vi "Get Data.vi"(7 "?":T1={"Input Data 1D"=[], "Channel Settings"={"Supply Voltage [Vdc]"=0.0, "Max Supply Current [Idc]"=0.0, "Settling Delay"=0.0, "Temp Criteria"=0.0, "Voltage Steps [Vrms]"=[0.0, 0.25, 0.5, 1.0, 1.95, 3.0, 3.9, 5.5], "User Notes"="", "Config Wave File Path"=path "C:/ASD Power Point Beta 32J/Waveforms/150HzSine5Second.wav", "Config Voltage [Vrms]"=0.0, "Channel Configuration List"={"Channel Configuration Cluster"={"Input"=enum."---", "Enable"=FALSE, "User Notes"="", "Voltage Range"=0.0, "Current Range"=2.5}, "Channel Configuration Cluster 2"={"Input"=enum."---", "Enable"=FALSE, "User Notes"="", "Voltage Range"=0.0, "Current Range"=2.5}, "Channel Configuration Cluster 3"={"Input"=enum."---", "Enable"=FALSE, "User Notes"="", "Voltage Range"=0.0, "Current Range"=2.5}, "Channel Configuration Cluster 4"={"Input"=enum."---", "Enable"=FALSE, "User Notes"="", "Voltage Range"=0.0, "Current Range"=2.5}, "Channel Configuration Cluster 5"={"Input"=enum."---", "Enable"=FALSE, "User Notes"="", "Voltage Range"=0.0, "Current Range"=2.5}, "Channel Configuration Cluster 6"={"Input"=enum."---", "Enable"=FALSE, "User Notes"="", "Voltage Range"=0.0, "Current Range"=2.5}, "Channel Configuration Cluster 7"={"Input"=enum."---", "Enable"=FALSE, "User Notes"="", "Voltage Range"=0.0, "Current Range"=2.5}, "Channel Configuration Cluster 8"={"Input"=enum."---", "Enable"=FALSE, "User Notes"="", "Voltage Range"=0.0, "Current Range"=2.5}, "Channel Configuration Cluster 9"={"Input"=enum."---", "Enable"=FALSE, "User Notes"="", "Voltage Range"=0.0, "Current Range"=2.5}, "Channel Configuration Cluster 10"={"Input"=enum."---", "Enable"=FALSE, "User Notes"="", "Voltage Range"=0.0, "Current Range"=2.5}, "Channel Configuration Cluster 11"={"Input"=enum."---", "Enable"=FALSE, "User Notes"="", "Voltage Range"=0.0, "Current Range"=2.5}, "Channel Configuration Cluster 12"={"Input"=enum."---", "Enable"=FALSE, "User Notes"="", "Voltage Range"=0.0, "Current Range"=2.5}, "Channel Configuration Cluster 13"={"Input"=enum."---", "Enable"=FALSE, "User Notes"="", "Voltage Range"=0.0, "Current Range"=2.5}, "Channel Configuration Cluster 14"={"Input"=enum."---", "Enable"=FALSE, "User Notes"="", "Voltage Range"=0.0, "Current Range"=2.5}, "Channel Configuration Cluster 15"={"Input"=enum."---", "Enable"=FALSE, "User Notes"="", "Voltage Range"=0.0, "Current Range"=2.5}, "Channel Configuration Cluster 16"={"Input"=enum."---", "Enable"=FALSE, "User Notes"="", "Voltage Range"=0.0, "Current Range"=2.5}, "Channel Configuration Cluster 17"={"Input"=enum."---", "Enable"=FALSE, "User Notes"="", "Voltage Range"=0.0, "Current Range"=2.5}}, "User Gains"={"Gain 1"=0.0, "Gain 2"=0.0, "Gain 3"=0.0, "Gain 4"=0.0, "Gain 5"=0.0, "Gain 6"=0.0}, "Gains"={"Gain 1"=0.0, "Gain 2"=0.0, "Gain 3"=0.0, "Gain 4"=0.0, "Gain 5"=0.0, "Gain 6"=0.0}, "Gain Array"={"Gain 1"=0.0, "Gain 2"=0.0, "Gain 3"=0.0, "Gain 4"=0.0, "Gain 5"=0.0, "Gain 6"=0.0, "Gain 7"=0.0, "Gain 8"=0.0, "Gain 9"=0.0, "Gain 10"=0.0, "Gain 11"=0.0, "Gain 12"=0.0, "Gain 13"=0.0, "Gain 14"=0.0, "Gain 15"=0.0, "Gain 16"=0.0, "Gain 17"=0.0}, "Wave File Path 1"=path "", "Wave File Path 2"=path "", "Wave File Path 3"=path "", "Wave File Path 4"=path "", "Range"=FALSE, "CF"=FALSE}, "Select Data"={"Vrms Data"=FALSE, "Vpkpk Data"=FALSE, "Irms Data"=FALSE, "Power Data"=FALSE, "Ipkpk Data"=FALSE, "Temp Data"=FALSE}, "Detailed Report ?"=FALSE, "Path Settings:"={"Template Path "=path "E:/L&T Projects/Bose ASD/Excel Template/ASD Template.xltx", "Report Path"=path "E:/L&T Projects/Bose ASD/excel Reports", "JPEG1 Path "=path "C:/Users/Public/Pictures/Sample Pictures/Hydrangeas.jpg", "JPEG2 Path"=path "C:/Users/Public/Pictures/Sample Pictures/Lighthouse.jpg"}, "Vrms_Sheet"=[], "Irms_Sheet"=[], "Power_Sheet"=[], "Vpk_Sheet"=[], "Ipk_Sheet"=[], "Vrms_Avg"=[], "Irms_Avg"=[], "Power_Avg"=[], "Vpk_Avg"=[], "Ipk_Avg"=[], "Report_Ref"=refnum, "User Name"="", "Temp_Sheet"=[]} {"Channel Settings"."Gain Array"."Gain 17" format="%.2f"; "Channel Settings"."Gain Array"."Gain 16" format="%.2f"; "Channel Settings"."Gain Array"."Gain 15" format="%.2f"; "Channel Settings"."Gain Array"."Gain 14" format="%.2f"; "Channel Settings"."Gain Array"."Gain 13" format="%.2f"; "Channel Settings"."Gain Array"."Gain 12" format="%.2f"; "Channel Settings"."Gain Array"."Gain 11" format="%.2f"; "Channel Settings"."Gain Array"."Gain 10" format="%.2f"; "Channel Settings"."Gain Array"."Gain 9" format="%.2f"; "Channel Settings"."Gain Array"."Gain 8" format="%.2f"; "Channel Settings"."Gain Array"."Gain 7" format="%.2f"; "Channel Settings"."Gain Array"."Gain 6" format="%.2f"; "Channel Settings"."Gain Array"."Gain 5" format="%.2f"; "Channel Settings"."Gain Array"."Gain 4" format="%.2f"; "Channel Settings"."Gain Array"."Gain 3" format="%.2f"; "Channel Settings"."Gain Array"."Gain 2" format="%.2f"; "Channel Settings"."Gain Array"."Gain 1" format="%.2f"; "Channel Settings"."Gains"."Gain 6" format="%.2f"; "Channel Settings"."Gains"."Gain 5" format="%.2f"; "Channel Settings"."Gains"."Gain 4" format="%.2f"; "Channel Settings"."Gains"."Gain 3" format="%.2f"; "Channel Settings"."Gains"."Gain 2" format="%.2f"; "Channel Settings"."Gains"."Gain 1" format="%.2f"; "Channel Settings"."User Gains"."Gain 6" format="%.2f"; "Channel Settings"."User Gains"."Gain 5" format="%.2f"; "Channel Settings"."User Gains"."Gain 4" format="%.2f"; "Channel Settings"."User Gains"."Gain 3" format="%.2f"; "Channel Settings"."User Gains"."Gain 2" format="%.2f"; "Channel Settings"."User Gains"."Gain 1" format="%.2f"; "Channel Settings"."Channel Configuration List"."Channel Configuration Cluster 17"."Current Range" items=["1 <500m>"=0.5, "2 <1>"=1.0, "5 <2.5>"=2.5, "10 <5>"=5.0, "20 <10>"=10.0, "50 <25>"=25.0]; "Channel Settings"."Channel Configuration List"."Channel Configuration Cluster 17"."Voltage Range" items=["1.5 <0.75>"=0.75, "3 <1.5>"=1.5, "6 <3>"=3.0, "10 <5>"=5.0, "15 <7.5>"=7.5, "30 <15>"=15.0, "60 <30>"=30.0, "100 <50>"=50.0, "150 <75>"=75.0, "300 <150>"=150.0, "600 <300>"=300.0, "1000 <500>"=500.0]; "Channel Settings"."Channel Configuration List"."Channel Configuration Cluster 16"."Current Range" items=["1 <500m>"=0.5, "2 <1>"=1.0, "5 <2.5>"=2.5, "10 <5>"=5.0, "20 <10>"=10.0, "50 <25>"=25.0]; "Channel Settings"."Channel Configuration List"."Channel Configuration Cluster 16"."Voltage Range" items=["1.5 <0.75>"=0.75, "3 <1.5>"=1.5, "6 <3>"=3.0, "10 <5>"=5.0, "15 <7.5>"=7.5, "30 <15>"=15.0, "60 <30>"=30.0, "100 <50>"=50.0, "150 <75>"=75.0, "300 <150>"=150.0, "600 <300>"=300.0, "1000 <500>"=500.0]; "Channel Settings"."Channel Configuration List"."Channel Configuration Cluster 15"."Current Range" items=["1 <500m>"=0.5, "2 <1>"=1.0, "5 <2.5>"=2.5, "10 <5>"=5.0, "20 <10>"=10.0, "50 <25>"=25.0]; "Channel Settings"."Channel Configuration List"."Channel Configuration Cluster 15"."Voltage Range" items=["1.5 <0.75>"=0.75, "3 <1.5>"=1.5, "6 <3>"=3.0, "10 <5>"=5.0, "15 <7.5>"=7.5, "30 <15>"=15.0, "60 <30>"=30.0, "100 <50>"=50.0, "150 <75>"=75.0, "300 <150>"=150.0, "600 <300>"=300.0, "1000 <500>"=500.0]; "Channel Settings"."Channel Configuration List"."Channel Configuration Cluster 14"."Current Range" items=["1 <500m>"=0.5, "2 <1>"=1.0, "5 <2.5>"=2.5, "10 <5>"=5.0, "20 <10>"=10.0, "50 <25>"=25.0]; "Channel Settings"."Channel Configuration List"."Channel Configuration Cluster 14"."Voltage Range" items=["1.5 <0.75>"=0.75, "3 <1.5>"=1.5, "6 <3>"=3.0, "10 <5>"=5.0, "15 <7.5>"=7.5, "30 <15>"=15.0, "60 <30>"=30.0, "100 <50>"=50.0, "150 <75>"=75.0, "300 <150>"=150.0, "600 <300>"=300.0, "1000 <500>"=500.0]; "Channel Settings"."Channel Configuration List"."Channel Configuration Cluster 13"."Current Range" items=["1 <500m>"=0.5, "2 <1>"=1.0, "5 <2.5>"=2.5, "10 <5>"=5.0, "20 <10>"=10.0, "50 <25>"=25.0]; "Channel Settings"."Channel Configuration List"."Channel Configuration Cluster 13"."Voltage Range" items=["1.5 <0.75>"=0.75, "3 <1.5>"=1.5, "6 <3>"=3.0, "10 <5>"=5.0, "15 <7.5>"=7.5, "30 <15>"=15.0, "60 <30>"=30.0, "100 <50>"=50.0, "150 <75>"=75.0, "300 <150>"=150.0, "600 <300>"=300.0, "1000 <500>"=500.0]; "Channel Settings"."Channel Configuration List"."Channel Configuration Cluster 12"."Current Range" items=["1 <500m>"=0.5, "2 <1>"=1.0, "5 <2.5>"=2.5, "10 <5>"=5.0, "20 <10>"=10.0, "50 <25>"=25.0]; "Channel Settings"."Channel Configuration List"."Channel Configuration Cluster 12"."Voltage Range" items=["1.5 <0.75>"=0.75, "3 <1.5>"=1.5, "6 <3>"=3.0, "10 <5>"=5.0, "15 <7.5>"=7.5, "30 <15>"=15.0, "60 <30>"=30.0, "100 <50>"=50.0, "150 <75>"=75.0, "300 <150>"=150.0, "600 <300>"=300.0, "1000 <500>"=500.0]; "Channel Settings"."Channel Configuration List"."Channel Configuration Cluster 11"."Current Range" items=["1 <500m>"=0.5, "2 <1>"=1.0, "5 <2.5>"=2.5, "10 <5>"=5.0, "20 <10>"=10.0, "50 <25>"=25.0]; "Channel Settings"."Channel Configuration List"."Channel Configuration Cluster 11"."Voltage Range" items=["1.5 <0.75>"=0.75, "3 <1.5>"=1.5, "6 <3>"=3.0, "10 <5>"=5.0, "15 <7.5>"=7.5, "30 <15>"=15.0, "60 <30>"=30.0, "100 <50>"=50.0, "150 <75>"=75.0, "300 <150>"=150.0, "600 <300>"=300.0, "1000 <500>"=500.0]; "Channel Settings"."Channel Configuration List"."Channel Configuration Cluster 10"."Current Range" items=["1 <500m>"=0.5, "2 <1>"=1.0, "5 <2.5>"=2.5, "10 <5>"=5.0, "20 <10>"=10.0, "50 <25>"=25.0]; "Channel Settings"."Channel Configuration List"."Channel Configuration Cluster 10"."Voltage Range" items=["1.5 <0.75>"=0.75, "3 <1.5>"=1.5, "6 <3>"=3.0, "10 <5>"=5.0, "15 <7.5>"=7.5, "30 <15>"=15.0, "60 <30>"=30.0, "100 <50>"=50.0, "150 <75>"=75.0, "300 <150>"=150.0, "600 <300>"=300.0, "1000 <500>"=500.0]; "Channel Settings"."Channel Configuration List"."Channel Configuration Cluster 9"."Voltage Range" items=["1.5 <0.75>"=0.75, "3 <1.5>"=1.5, "6 <3>"=3.0, "10 <5>"=5.0, "15 <7.5>"=7.5, "30 <15>"=15.0, "60 <30>"=30.0, "100 <50>"=50.0, "150 <75>"=75.0, "300 <150>"=150.0, "600 <300>"=300.0, "1000 <500>"=500.0]; "Channel Settings"."Channel Configuration List"."Channel Configuration Cluster 9"."Current Range" items=["10m <5m>"=0.005, "20m <10m>"=0.01, "50m <25m>"=0.025, "100m <50m>"=0.05, "200m <100m>"=0.1, "500m <250m>"=0.25, "1 <500m>"=0.5, "2 <1>"=1.0, "5 <2.5>"=2.5]; "Channel Settings"."Channel Configuration List"."Channel Configuration Cluster 8"."Voltage Range" items=["1.5 <0.75>"=0.75, "3 <1.5>"=1.5, "6 <3>"=3.0, "10 <5>"=5.0, "15 <7.5>"=7.5, "30 <15>"=15.0, "60 <30>"=30.0, "100 <50>"=50.0, "150 <75>"=75.0, "300 <150>"=150.0, "600 <300>"=300.0, "1000 <500>"=500.0]; "Channel Settings"."Channel Configuration List"."Channel Configuration Cluster 8"."Current Range" items=["10m <5m>"=0.005, "20m <10m>"=0.01, "50m <25m>"=0.025, "100m <50m>"=0.05, "200m <100m>"=0.1, "500m <250m>"=0.25, "1 <500m>"=0.5, "2 <1>"=1.0, "5 <2.5>"=2.5]; "Channel Settings"."Channel Configuration List"."Channel Configuration Cluster 7"."Voltage Range" items=["1.5 <0.75>"=0.75, "3 <1.5>"=1.5, "6 <3>"=3.0, "10 <5>"=5.0, "15 <7.5>"=7.5, "30 <15>"=15.0, "60 <30>"=30.0, "100 <50>"=50.0, "150 <75>"=75.0, "300 <150>"=150.0, "600 <300>"=300.0, "1000 <500>"=500.0]; "Channel Settings"."Channel Configuration List"."Channel Configuration Cluster 7"."Current Range" items=["10m <5m>"=0.005, "20m <10m>"=0.01, "50m <25m>"=0.025, "100m <50m>"=0.05, "200m <100m>"=0.1, "500m <250m>"=0.25, "1 <500m>"=0.5, "2 <1>"=1.0, "5 <2.5>"=2.5]; "Channel Settings"."Channel Configuration List"."Channel Configuration Cluster 6"."Voltage Range" items=["1.5 <0.75>"=0.75, "3 <1.5>"=1.5, "6 <3>"=3.0, "10 <5>"=5.0, "15 <7.5>"=7.5, "30 <15>"=15.0, "60 <30>"=30.0, "100 <50>"=50.0, "150 <75>"=75.0, "300 <150>"=150.0, "600 <300>"=300.0, "1000 <500>"=500.0]; "Channel Settings"."Channel Configuration List"."Channel Configuration Cluster 6"."Current Range" items=["10m <5m>"=0.005, "20m <10m>"=0.01, "50m <25m>"=0.025, "100m <50m>"=0.05, "200m <100m>"=0.1, "500m <250m>"=0.25, "1 <500m>"=0.5, "2 <1>"=1.0, "5 <2.5>"=2.5]; "Channel Settings"."Channel Configuration List"."Channel Configuration Cluster 5"."Voltage Range" items=["1.5 <0.75>"=0.75, "3 <1.5>"=1.5, "6 <3>"=3.0, "10 <5>"=5.0, "15 <7.5>"=7.5, "30 <15>"=15.0, "60 <30>"=30.0, "100 <50>"=50.0, "150 <75>"=75.0, "300 <150>"=150.0, "600 <300>"=300.0, "1000 <500>"=500.0]; "Channel Settings"."Channel Configuration List"."Channel Configuration Cluster 5"."Current Range" items=["10m <5m>"=0.005, "20m <10m>"=0.01, "50m <25m>"=0.025, "100m <50m>"=0.05, "200m <100m>"=0.1, "500m <250m>"=0.25, "1 <500m>"=0.5, "2 <1>"=1.0, "5 <2.5>"=2.5]; "Channel Settings"."Channel Configuration List"."Channel Configuration Cluster 4"."Voltage Range" items=["1.5 <0.75>"=0.75, "3 <1.5>"=1.5, "6 <3>"=3.0, "10 <5>"=5.0, "15 <7.5>"=7.5, "30 <15>"=15.0, "60 <30>"=30.0, "100 <50>"=50.0, "150 <75>"=75.0, "300 <150>"=150.0, "600 <300>"=300.0, "1000 <500>"=500.0]; "Channel Settings"."Channel Configuration List"."Channel Configuration Cluster 4"."Current Range" items=["10m <5m>"=0.005, "20m <10m>"=0.01, "50m <25m>"=0.025, "100m <50m>"=0.05, "200m <100m>"=0.1, "500m <250m>"=0.25, "1 <500m>"=0.5, "2 <1>"=1.0, "5 <2.5>"=2.5]; "Channel Settings"."Channel Configuration List"."Channel Configuration Cluster 3"."Voltage Range" items=["1.5 <0.75>"=0.75, "3 <1.5>"=1.5, "6 <3>"=3.0, "10 <5>"=5.0, "15 <7.5>"=7.5, "30 <15>"=15.0, "60 <30>"=30.0, "100 <50>"=50.0, "150 <75>"=75.0, "300 <150>"=150.0, "600 <300>"=300.0, "1000 <500>"=500.0]; "Channel Settings"."Channel Configuration List"."Channel Configuration Cluster 3"."Current Range" items=["10m <5m>"=0.005, "20m <10m>"=0.01, "50m <25m>"=0.025, "100m <50m>"=0.05, "200m <100m>"=0.1, "500m <250m>"=0.25, "1 <500m>"=0.5, "2 <1>"=1.0, "5 <2.5>"=2.5]; "Channel Settings"."Channel Configuration List"."Channel Configuration Cluster 2"."Voltage Range" items=["1.5 <0.75>"=0.75, "3 <1.5>"=1.5, "6 <3>"=3.0, "10 <5>"=5.0, "15 <7.5>"=7.5, "30 <15>"=15.0, "60 <30>"=30.0, "100 <50>"=50.0, "150 <75>"=75.0, "300 <150>"=150.0, "600 <300>"=300.0, "1000 <500>"=500.0]; "Channel Settings"."Channel Configuration List"."Channel Configuration Cluster 2"."Current Range" items=["10m <5m>"=0.005, "20m <10m>"=0.01, "50m <25m>"=0.025, "100m <50m>"=0.05, "200m <100m>"=0.1, "500m <250m>"=0.25, "1 <500m>"=0.5, "2 <1>"=1.0, "5 <2.5>"=2.5]; "Channel Settings"."Channel Configuration List"."Channel Configuration Cluster"."Voltage Range" items=["1.5 <0.75>"=0.75, "3 <1.5>"=1.5, "6 <3>"=3.0, "10 <5>"=5.0, "15 <7.5>"=7.5, "30 <15>"=15.0, "60 <30>"=30.0, "100 <50>"=50.0, "150 <75>"=75.0, "300 <150>"=150.0, "600 <300>"=300.0, "1000 <500>"=500.0]; "Channel Settings"."Channel Configuration List"."Channel Configuration Cluster"."Current Range" items=["10m <5m>"=0.005, "20m <10m>"=0.01, "50m <25m>"=0.025, "100m <50m>"=0.05, "200m <100m>"=0.1, "500m <250m>"=0.25, "1 <500m>"=0.5, "2 <1>"=1.0, "5 <2.5>"=2.5]; "Channel Settings"."Settling Delay" min=0.0 format="%<%H:%M:%S>t"; "Input Data 1D"."WT1800 Averages"."Vrms" format="%.3f"; "Input Data 1D"."WT1800 Averages"."Irms" format="%.3f"; "Input Data 1D"."WT1800 Averages"."Power" format="%.3f"; "Input Data 1D"."WT1800 Averages"."Vpkpk" format="%.3f"; "Input Data 1D"."WT1800 Averages"."Ipkpk" format="%.3f"; "Input Data 1D"."WT1800 Measurements"."Vrms" format="%.3f"; "Input Data 1D"."WT1800 Measurements"."Irms" format="%.3f"; "Input Data 1D"."WT1800 Measurements"."Power" format="%.3f"; "Input Data 1D"."WT1800 Measurements"."Vpkpk" format="%.3f"; "Input Data 1D"."WT1800 Measurements"."Ipkpk" format="%.3f"; "Input Data 1D"."DSA Averages"."Vrms" format="%.3f"; "Input Data 1D"."DSA Averages"."Vdc" format="%.3f"; "Input Data 1D"."DSA Averages"."Vpk+" format="%.3f"; "Input Data 1D"."DSA Averages"."Vpk-" format="%.3f"; "Input Data 1D"."DSA Averages"."Vpkpk" format="%.3f"; "Input Data 1D"."DSA Measurements"."Vrms" format="%.3f"; "Input Data 1D"."DSA Measurements"."Vdc" format="%.3f"; "Input Data 1D"."DSA Measurements"."Vpk+" format="%.3f"; "Input Data 1D"."DSA Measurements"."Vpk-" format="%.3f"; "Input Data 1D"."DSA Measurements"."Vpkpk" format="%.3f"}, 8 "error in":errorcluster) -> (0 "error out":errorcluster, 5 "output cluster":T1={"Input Data 1D"=[], "Channel Settings"={"Supply Voltage [Vdc]"=0.0, "Max Supply Current [Idc]"=0.0, "Settling Delay"=0.0, "Temp Criteria"=0.0, "Voltage Steps [Vrms]"=[0.0, 0.25, 0.5, 1.0, 1.95, 3.0, 3.9, 5.5], "User Notes"="", "Config Wave File Path"=path "C:/ASD Power Point Beta 32J/Waveforms/150HzSine5Second.wav", "Config Voltage [Vrms]"=0.0, "Channel Configuration List"={"Channel Configuration Cluster"={"Input"=enum."---", "Enable"=FALSE, "User Notes"="", "Voltage Range"=0.0, "Current Range"=2.5}, "Channel Configuration Cluster 2"={"Input"=enum."---", "Enable"=FALSE, "User Notes"="", "Voltage Range"=0.0, "Current Range"=2.5}, "Channel Configuration Cluster 3"={"Input"=enum."---", "Enable"=FALSE, "User Notes"="", "Voltage Range"=0.0, "Current Range"=2.5}, "Channel Configuration Cluster 4"={"Input"=enum."---", "Enable"=FALSE, "User Notes"="", "Voltage Range"=0.0, "Current Range"=2.5}, "Channel Configuration Cluster 5"={"Input"=enum."---", "Enable"=FALSE, "User Notes"="", "Voltage Range"=0.0, "Current Range"=2.5}, "Channel Configuration Cluster 6"={"Input"=enum."---", "Enable"=FALSE, "User Notes"="", "Voltage Range"=0.0, "Current Range"=2.5}, "Channel Configuration Cluster 7"={"Input"=enum."---", "Enable"=FALSE, "User Notes"="", "Voltage Range"=0.0, "Current Range"=2.5}, "Channel Configuration Cluster 8"={"Input"=enum."---", "Enable"=FALSE, "User Notes"="", "Voltage Range"=0.0, "Current Range"=2.5}, "Channel Configuration Cluster 9"={"Input"=enum."---", "Enable"=FALSE, "User Notes"="", "Voltage Range"=0.0, "Current Range"=2.5}, "Channel Configuration Cluster 10"={"Input"=enum."---", "Enable"=FALSE, "User Notes"="", "Voltage Range"=0.0, "Current Range"=2.5}, "Channel Configuration Cluster 11"={"Input"=enum."---", "Enable"=FALSE, "User Notes"="", "Voltage Range"=0.0, "Current Range"=2.5}, "Channel Configuration Cluster 12"={"Input"=enum."---", "Enable"=FALSE, "User Notes"="", "Voltage Range"=0.0, "Current Range"=2.5}, "Channel Configuration Cluster 13"={"Input"=enum."---", "Enable"=FALSE, "User Notes"="", "Voltage Range"=0.0, "Current Range"=2.5}, "Channel Configuration Cluster 14"={"Input"=enum."---", "Enable"=FALSE, "User Notes"="", "Voltage Range"=0.0, "Current Range"=2.5}, "Channel Configuration Cluster 15"={"Input"=enum."---", "Enable"=FALSE, "User Notes"="", "Voltage Range"=0.0, "Current Range"=2.5}, "Channel Configuration Cluster 16"={"Input"=enum."---", "Enable"=FALSE, "User Notes"="", "Voltage Range"=0.0, "Current Range"=2.5}, "Channel Configuration Cluster 17"={"Input"=enum."---", "Enable"=FALSE, "User Notes"="", "Voltage Range"=0.0, "Current Range"=2.5}}, "User Gains"={"Gain 1"=0.0, "Gain 2"=0.0, "Gain 3"=0.0, "Gain 4"=0.0, "Gain 5"=0.0, "Gain 6"=0.0}, "Gains"={"Gain 1"=0.0, "Gain 2"=0.0, "Gain 3"=0.0, "Gain 4"=0.0, "Gain 5"=0.0, "Gain 6"=0.0}, "Gain Array"={"Gain 1"=0.0, "Gain 2"=0.0, "Gain 3"=0.0, "Gain 4"=0.0, "Gain 5"=0.0, "Gain 6"=0.0, "Gain 7"=0.0, "Gain 8"=0.0, "Gain 9"=0.0, "Gain 10"=0.0, "Gain 11"=0.0, "Gain 12"=0.0, "Gain 13"=0.0, "Gain 14"=0.0, "Gain 15"=0.0, "Gain 16"=0.0, "Gain 17"=0.0}, "Wave File Path 1"=path "", "Wave File Path 2"=path "", "Wave File Path 3"=path "", "Wave File Path 4"=path "", "Range"=FALSE, "CF"=FALSE}, "Select Data"={"Vrms Data"=FALSE, "Vpkpk Data"=FALSE, "Irms Data"=FALSE, "Power Data"=FALSE, "Ipkpk Data"=FALSE, "Temp Data"=FALSE}, "Detailed Report ?"=FALSE, "Path Settings:"={"Template Path "=path "E:/L&T Projects/Bose ASD/Excel Template/ASD Template.xltx", "Report Path"=path "E:/L&T Projects/Bose ASD/excel Reports", "JPEG1 Path "=path "C:/Users/Public/Pictures/Sample Pictures/Hydrangeas.jpg", "JPEG2 Path"=path "C:/Users/Public/Pictures/Sample Pictures/Lighthouse.jpg"}, "Vrms_Sheet"=[], "Irms_Sheet"=[], "Power_Sheet"=[], "Vpk_Sheet"=[], "Ipk_Sheet"=[], "Vrms_Avg"=[], "Irms_Avg"=[], "Power_Avg"=[], "Vpk_Avg"=[], "Ipk_Avg"=[], "Report_Ref"=refnum, "User Name"="", "Temp_Sheet"=[]} {"Channel Settings"."Gain Array"."Gain 17" format="%.2f"; "Channel Settings"."Gain Array"."Gain 16" format="%.2f"; "Channel Settings"."Gain Array"."Gain 15" format="%.2f"; "Channel Settings"."Gain Array"."Gain 14" format="%.2f"; "Channel Settings"."Gain Array"."Gain 13" format="%.2f"; "Channel Settings"."Gain Array"."Gain 12" format="%.2f"; "Channel Settings"."Gain Array"."Gain 11" format="%.2f"; "Channel Settings"."Gain Array"."Gain 10" format="%.2f"; "Channel Settings"."Gain Array"."Gain 9" format="%.2f"; "Channel Settings"."Gain Array"."Gain 8" format="%.2f"; "Channel Settings"."Gain Array"."Gain 7" format="%.2f"; "Channel Settings"."Gain Array"."Gain 6" format="%.2f"; "Channel Settings"."Gain Array"."Gain 5" format="%.2f"; "Channel Settings"."Gain Array"."Gain 4" format="%.2f"; "Channel Settings"."Gain Array"."Gain 3" format="%.2f"; "Channel Settings"."Gain Array"."Gain 2" format="%.2f"; "Channel Settings"."Gain Array"."Gain 1" format="%.2f"; "Channel Settings"."Gains"."Gain 6" format="%.2f"; "Channel Settings"."Gains"."Gain 5" format="%.2f"; "Channel Settings"."Gains"."Gain 4" format="%.2f"; "Channel Settings"."Gains"."Gain 3" format="%.2f"; "Channel Settings"."Gains"."Gain 2" format="%.2f"; "Channel Settings"."Gains"."Gain 1" format="%.2f"; "Channel Settings"."User Gains"."Gain 6" format="%.2f"; "Channel Settings"."User Gains"."Gain 5" format="%.2f"; "Channel Settings"."User Gains"."Gain 4" format="%.2f"; "Channel Settings"."User Gains"."Gain 3" format="%.2f"; "Channel Settings"."User Gains"."Gain 2" format="%.2f"; "Channel Settings"."User Gains"."Gain 1" format="%.2f"; "Channel Settings"."Channel Configuration List"."Channel Configuration Cluster 17"."Current Range" items=["1 <500m>"=0.5, "2 <1>"=1.0, "5 <2.5>"=2.5, "10 <5>"=5.0, "20 <10>"=10.0, "50 <25>"=25.0]; "Channel Settings"."Channel Configuration List"."Channel Configuration Cluster 17"."Voltage Range" items=["1.5 <0.75>"=0.75, "3 <1.5>"=1.5, "6 <3>"=3.0, "10 <5>"=5.0, "15 <7.5>"=7.5, "30 <15>"=15.0, "60 <30>"=30.0, "100 <50>"=50.0, "150 <75>"=75.0, "300 <150>"=150.0, "600 <300>"=300.0, "1000 <500>"=500.0]; "Channel Settings"."Channel Configuration List"."Channel Configuration Cluster 16"."Current Range" items=["1 <500m>"=0.5, "2 <1>"=1.0, "5 <2.5>"=2.5, "10 <5>"=5.0, "20 <10>"=10.0, "50 <25>"=25.0]; "Channel Settings"."Channel Configuration List"."Channel Configuration Cluster 16"."Voltage Range" items=["1.5 <0.75>"=0.75, "3 <1.5>"=1.5, "6 <3>"=3.0, "10 <5>"=5.0, "15 <7.5>"=7.5, "30 <15>"=15.0, "60 <30>"=30.0, "100 <50>"=50.0, "150 <75>"=75.0, "300 <150>"=150.0, "600 <300>"=300.0, "1000 <500>"=500.0]; "Channel Settings"."Channel Configuration List"."Channel Configuration Cluster 15"."Current Range" items=["1 <500m>"=0.5, "2 <1>"=1.0, "5 <2.5>"=2.5, "10 <5>"=5.0, "20 <10>"=10.0, "50 <25>"=25.0]; "Channel Settings"."Channel Configuration List"."Channel Configuration Cluster 15"."Voltage Range" items=["1.5 <0.75>"=0.75, "3 <1.5>"=1.5, "6 <3>"=3.0, "10 <5>"=5.0, "15 <7.5>"=7.5, "30 <15>"=15.0, "60 <30>"=30.0, "100 <50>"=50.0, "150 <75>"=75.0, "300 <150>"=150.0, "600 <300>"=300.0, "1000 <500>"=500.0]; "Channel Settings"."Channel Configuration List"."Channel Configuration Cluster 14"."Current Range" items=["1 <500m>"=0.5, "2 <1>"=1.0, "5 <2.5>"=2.5, "10 <5>"=5.0, "20 <10>"=10.0, "50 <25>"=25.0]; "Channel Settings"."Channel Configuration List"."Channel Configuration Cluster 14"."Voltage Range" items=["1.5 <0.75>"=0.75, "3 <1.5>"=1.5, "6 <3>"=3.0, "10 <5>"=5.0, "15 <7.5>"=7.5, "30 <15>"=15.0, "60 <30>"=30.0, "100 <50>"=50.0, "150 <75>"=75.0, "300 <150>"=150.0, "600 <300>"=300.0, "1000 <500>"=500.0]; "Channel Settings"."Channel Configuration List"."Channel Configuration Cluster 13"."Current Range" items=["1 <500m>"=0.5, "2 <1>"=1.0, "5 <2.5>"=2.5, "10 <5>"=5.0, "20 <10>"=10.0, "50 <25>"=25.0]; "Channel Settings"."Channel Configuration List"."Channel Configuration Cluster 13"."Voltage Range" items=["1.5 <0.75>"=0.75, "3 <1.5>"=1.5, "6 <3>"=3.0, "10 <5>"=5.0, "15 <7.5>"=7.5, "30 <15>"=15.0, "60 <30>"=30.0, "100 <50>"=50.0, "150 <75>"=75.0, "300 <150>"=150.0, "600 <300>"=300.0, "1000 <500>"=500.0]; "Channel Settings"."Channel Configuration List"."Channel Configuration Cluster 12"."Current Range" items=["1 <500m>"=0.5, "2 <1>"=1.0, "5 <2.5>"=2.5, "10 <5>"=5.0, "20 <10>"=10.0, "50 <25>"=25.0]; "Channel Settings"."Channel Configuration List"."Channel Configuration Cluster 12"."Voltage Range" items=["1.5 <0.75>"=0.75, "3 <1.5>"=1.5, "6 <3>"=3.0, "10 <5>"=5.0, "15 <7.5>"=7.5, "30 <15>"=15.0, "60 <30>"=30.0, "100 <50>"=50.0, "150 <75>"=75.0, "300 <150>"=150.0, "600 <300>"=300.0, "1000 <500>"=500.0]; "Channel Settings"."Channel Configuration List"."Channel Configuration Cluster 11"."Current Range" items=["1 <500m>"=0.5, "2 <1>"=1.0, "5 <2.5>"=2.5, "10 <5>"=5.0, "20 <10>"=10.0, "50 <25>"=25.0]; "Channel Settings"."Channel Configuration List"."Channel Configuration Cluster 11"."Voltage Range" items=["1.5 <0.75>"=0.75, "3 <1.5>"=1.5, "6 <3>"=3.0, "10 <5>"=5.0, "15 <7.5>"=7.5, "30 <15>"=15.0, "60 <30>"=30.0, "100 <50>"=50.0, "150 <75>"=75.0, "300 <150>"=150.0, "600 <300>"=300.0, "1000 <500>"=500.0]; "Channel Settings"."Channel Configuration List"."Channel Configuration Cluster 10"."Current Range" items=["1 <500m>"=0.5, "2 <1>"=1.0, "5 <2.5>"=2.5, "10 <5>"=5.0, "20 <10>"=10.0, "50 <25>"=25.0]; "Channel Settings"."Channel Configuration List"."Channel Configuration Cluster 10"."Voltage Range" items=["1.5 <0.75>"=0.75, "3 <1.5>"=1.5, "6 <3>"=3.0, "10 <5>"=5.0, "15 <7.5>"=7.5, "30 <15>"=15.0, "60 <30>"=30.0, "100 <50>"=50.0, "150 <75>"=75.0, "300 <150>"=150.0, "600 <300>"=300.0, "1000 <500>"=500.0]; "Channel Settings"."Channel Configuration List"."Channel Configuration Cluster 9"."Voltage Range" items=["1.5 <0.75>"=0.75, "3 <1.5>"=1.5, "6 <3>"=3.0, "10 <5>"=5.0, "15 <7.5>"=7.5, "30 <15>"=15.0, "60 <30>"=30.0, "100 <50>"=50.0, "150 <75>"=75.0, "300 <150>"=150.0, "600 <300>"=300.0, "1000 <500>"=500.0]; "Channel Settings"."Channel Configuration List"."Channel Configuration Cluster 9"."Current Range" items=["10m <5m>"=0.005, "20m <10m>"=0.01, "50m <25m>"=0.025, "100m <50m>"=0.05, "200m <100m>"=0.1, "500m <250m>"=0.25, "1 <500m>"=0.5, "2 <1>"=1.0, "5 <2.5>"=2.5]; "Channel Settings"."Channel Configuration List"."Channel Configuration Cluster 8"."Voltage Range" items=["1.5 <0.75>"=0.75, "3 <1.5>"=1.5, "6 <3>"=3.0, "10 <5>"=5.0, "15 <7.5>"=7.5, "30 <15>"=15.0, "60 <30>"=30.0, "100 <50>"=50.0, "150 <75>"=75.0, "300 <150>"=150.0, "600 <300>"=300.0, "1000 <500>"=500.0]; "Channel Settings"."Channel Configuration List"."Channel Configuration Cluster 8"."Current Range" items=["10m <5m>"=0.005, "20m <10m>"=0.01, "50m <25m>"=0.025, "100m <50m>"=0.05, "200m <100m>"=0.1, "500m <250m>"=0.25, "1 <500m>"=0.5, "2 <1>"=1.0, "5 <2.5>"=2.5]; "Channel Settings"."Channel Configuration List"."Channel Configuration Cluster 7"."Voltage Range" items=["1.5 <0.75>"=0.75, "3 <1.5>"=1.5, "6 <3>"=3.0, "10 <5>"=5.0, "15 <7.5>"=7.5, "30 <15>"=15.0, "60 <30>"=30.0, "100 <50>"=50.0, "150 <75>"=75.0, "300 <150>"=150.0, "600 <300>"=300.0, "1000 <500>"=500.0]; "Channel Settings"."Channel Configuration List"."Channel Configuration Cluster 7"."Current Range" items=["10m <5m>"=0.005, "20m <10m>"=0.01, "50m <25m>"=0.025, "100m <50m>"=0.05, "200m <100m>"=0.1, "500m <250m>"=0.25, "1 <500m>"=0.5, "2 <1>"=1.0, "5 <2.5>"=2.5]; "Channel Settings"."Channel Configuration List"."Channel Configuration Cluster 6"."Voltage Range" items=["1.5 <0.75>"=0.75, "3 <1.5>"=1.5, "6 <3>"=3.0, "10 <5>"=5.0, "15 <7.5>"=7.5, "30 <15>"=15.0, "60 <30>"=30.0, "100 <50>"=50.0, "150 <75>"=75.0, "300 <150>"=150.0, "600 <300>"=300.0, "1000 <500>"=500.0]; "Channel Settings"."Channel Configuration List"."Channel Configuration Cluster 6"."Current Range" items=["10m <5m>"=0.005, "20m <10m>"=0.01, "50m <25m>"=0.025, "100m <50m>"=0.05, "200m <100m>"=0.1, "500m <250m>"=0.25, "1 <500m>"=0.5, "2 <1>"=1.0, "5 <2.5>"=2.5]; "Channel Settings"."Channel Configuration List"."Channel Configuration Cluster 5"."Voltage Range" items=["1.5 <0.75>"=0.75, "3 <1.5>"=1.5, "6 <3>"=3.0, "10 <5>"=5.0, "15 <7.5>"=7.5, "30 <15>"=15.0, "60 <30>"=30.0, "100 <50>"=50.0, "150 <75>"=75.0, "300 <150>"=150.0, "600 <300>"=300.0, "1000 <500>"=500.0]; "Channel Settings"."Channel Configuration List"."Channel Configuration Cluster 5"."Current Range" items=["10m <5m>"=0.005, "20m <10m>"=0.01, "50m <25m>"=0.025, "100m <50m>"=0.05, "200m <100m>"=0.1, "500m <250m>"=0.25, "1 <500m>"=0.5, "2 <1>"=1.0, "5 <2.5>"=2.5]; "Channel Settings"."Channel Configuration List"."Channel Configuration Cluster 4"."Voltage Range" items=["1.5 <0.75>"=0.75, "3 <1.5>"=1.5, "6 <3>"=3.0, "10 <5>"=5.0, "15 <7.5>"=7.5, "30 <15>"=15.0, "60 <30>"=30.0, "100 <50>"=50.0, "150 <75>"=75.0, "300 <150>"=150.0, "600 <300>"=300.0, "1000 <500>"=500.0]; "Channel Settings"."Channel Configuration List"."Channel Configuration Cluster 4"."Current Range" items=["10m <5m>"=0.005, "20m <10m>"=0.01, "50m <25m>"=0.025, "100m <50m>"=0.05, "200m <100m>"=0.1, "500m <250m>"=0.25, "1 <500m>"=0.5, "2 <1>"=1.0, "5 <2.5>"=2.5]; "Channel Settings"."Channel Configuration List"."Channel Configuration Cluster 3"."Voltage Range" items=["1.5 <0.75>"=0.75, "3 <1.5>"=1.5, "6 <3>"=3.0, "10 <5>"=5.0, "15 <7.5>"=7.5, "30 <15>"=15.0, "60 <30>"=30.0, "100 <50>"=50.0, "150 <75>"=75.0, "300 <150>"=150.0, "600 <300>"=300.0, "1000 <500>"=500.0]; "Channel Settings"."Channel Configuration List"."Channel Configuration Cluster 3"."Current Range" items=["10m <5m>"=0.005, "20m <10m>"=0.01, "50m <25m>"=0.025, "100m <50m>"=0.05, "200m <100m>"=0.1, "500m <250m>"=0.25, "1 <500m>"=0.5, "2 <1>"=1.0, "5 <2.5>"=2.5]; "Channel Settings"."Channel Configuration List"."Channel Configuration Cluster 2"."Voltage Range" items=["1.5 <0.75>"=0.75, "3 <1.5>"=1.5, "6 <3>"=3.0, "10 <5>"=5.0, "15 <7.5>"=7.5, "30 <15>"=15.0, "60 <30>"=30.0, "100 <50>"=50.0, "150 <75>"=75.0, "300 <150>"=150.0, "600 <300>"=300.0, "1000 <500>"=500.0]; "Channel Settings"."Channel Configuration List"."Channel Configuration Cluster 2"."Current Range" items=["10m <5m>"=0.005, "20m <10m>"=0.01, "50m <25m>"=0.025, "100m <50m>"=0.05, "200m <100m>"=0.1, "500m <250m>"=0.25, "1 <500m>"=0.5, "2 <1>"=1.0, "5 <2.5>"=2.5]; "Channel Settings"."Channel Configuration List"."Channel Configuration Cluster"."Voltage Range" items=["1.5 <0.75>"=0.75, "3 <1.5>"=1.5, "6 <3>"=3.0, "10 <5>"=5.0, "15 <7.5>"=7.5, "30 <15>"=15.0, "60 <30>"=30.0, "100 <50>"=50.0, "150 <75>"=75.0, "300 <150>"=150.0, "600 <300>"=300.0, "1000 <500>"=500.0]; "Channel Settings"."Channel Configuration List"."Channel Configuration Cluster"."Current Range" items=["10m <5m>"=0.005, "20m <10m>"=0.01, "50m <25m>"=0.025, "100m <50m>"=0.05, "200m <100m>"=0.1, "500m <250m>"=0.25, "1 <500m>"=0.5, "2 <1>"=1.0, "5 <2.5>"=2.5]; "Channel Settings"."Settling Delay" min=0.0 format="%<%H:%M:%S>t"; "Input Data 1D"."WT1800 Averages"."Vrms" format="%.3f"; "Input Data 1D"."WT1800 Averages"."Irms" format="%.3f"; "Input Data 1D"."WT1800 Averages"."Power" format="%.3f"; "Input Data 1D"."WT1800 Averages"."Vpkpk" format="%.3f"; "Input Data 1D"."WT1800 Averages"."Ipkpk" format="%.3f"; "Input Data 1D"."WT1800 Measurements"."Vrms" format="%.3f"; "Input Data 1D"."WT1800 Measurements"."Irms" format="%.3f"; "Input Data 1D"."WT1800 Measurements"."Power" format="%.3f"; "Input Data 1D"."WT1800 Measurements"."Vpkpk" format="%.3f"; "Input Data 1D"."WT1800 Measurements"."Ipkpk" format="%.3f"; "Input Data 1D"."DSA Averages"."Vrms" format="%.3f"; "Input Data 1D"."DSA Averages"."Vdc" format="%.3f"; "Input Data 1D"."DSA Averages"."Vpk+" format="%.3f"; "Input Data 1D"."DSA Averages"."Vpk-" format="%.3f"; "Input Data 1D"."DSA Averages"."Vpkpk" format="%.3f"; "Input Data 1D"."DSA Measurements"."Vrms" format="%.3f"; "Input Data 1D"."DSA Measurements"."Vdc" format="%.3f"; "Input Data 1D"."DSA Measurements"."Vpk+" format="%.3f"; "Input Data 1D"."DSA Measurements"."Vpk-" format="%.3f"; "Input Data 1D"."DSA Measurements"."Vpkpk" format="%.3f"})   [LabVIEW 2021]
uses:
  Datalog Controls/Data.ctl
  <vilib>/Utility/NIReport.llb/NI_report.lvclass
  Controls/Datalog Cluster Array.ctl
  Controls/Datalog Bundle Control.ctl
  Controls/WT1800 Functions.ctl
  Controls/WT1800 Measurements.ctl
  Controls/WT1800 Readings.ctl
  Controls/DSA Functions.ctl
  Controls/DSA Measurements.ctl
  Controls/DSA Readings.ctl
  Controls/Settings Control.ctl
  Controls/Channel Configuration List.ctl
  Controls/Channel Configuration Cluster.ctl
  Controls/Channel Configuration Cluster High Current.ctl
  Controls/Gain Averages.ctl
  Controls/Gain Array.ctl
  Datalog Controls/Select_Data.ctl
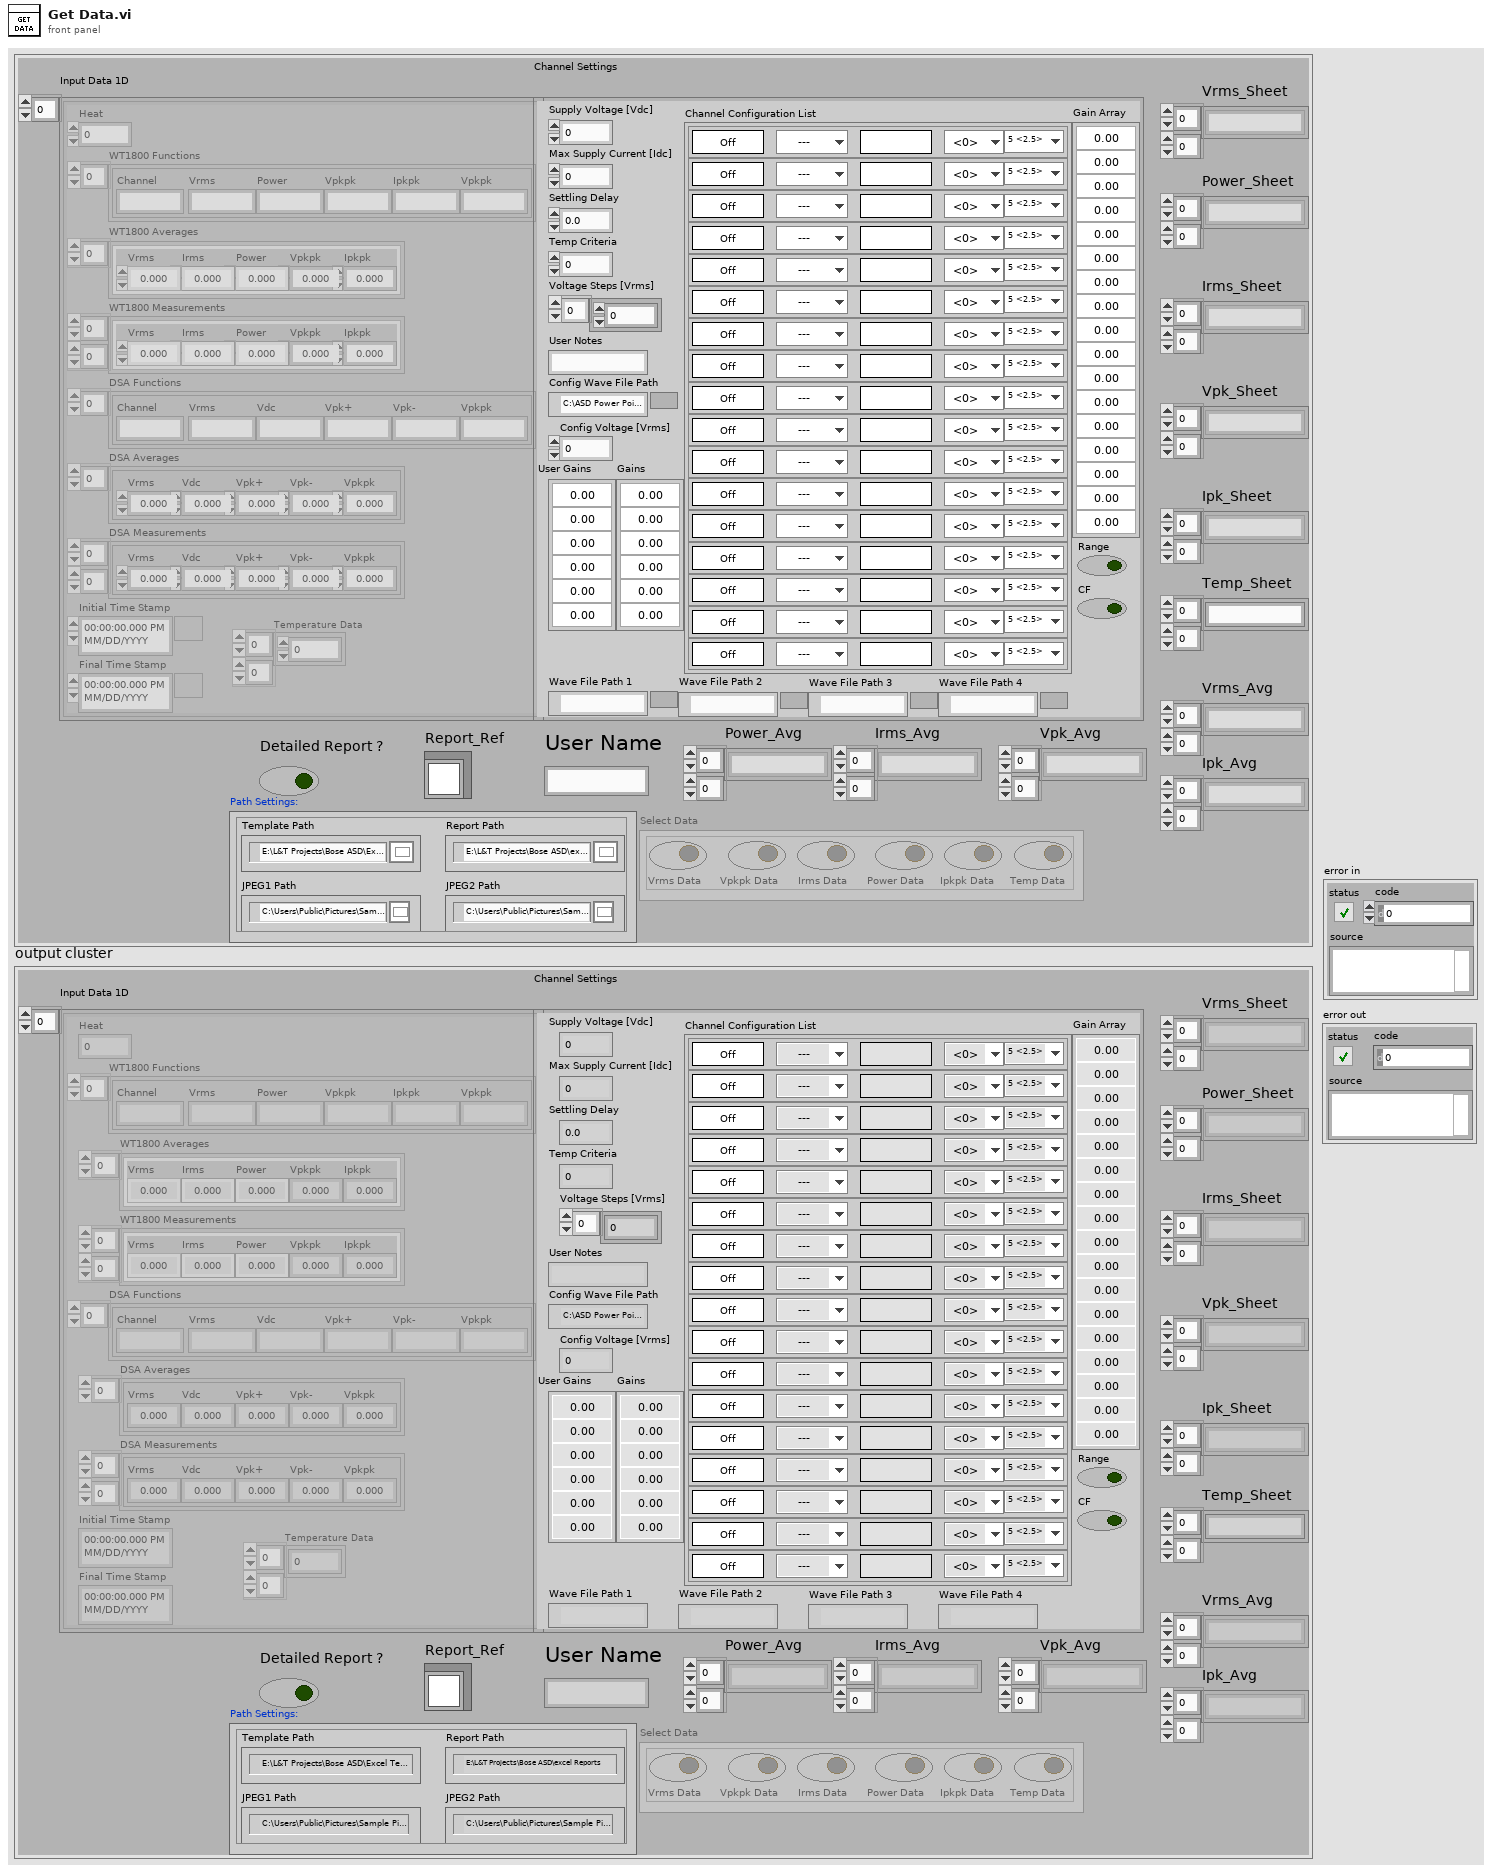
[diagram p1: front panel]
types:
  T1 = typedef "Data.ctl" = cluster{"Input Data 1D":T2, "Channel Settings":T10, "Select Data":T16, "Detailed Report ?":bool, "Path Settings:":cluster{"Template Path ":path, "Report Path":path, "JPEG1 Path ":path, "JPEG2 Path":path}, "Vrms_Sheet":string[][], "Irms_Sheet":string[][], "Power_Sheet":string[][], "Vpk_Sheet":string[][], "Ipk_Sheet":string[][], "Vrms_Avg":string[][], "Irms_Avg":string[][], "Power_Avg":string[][], "Vpk_Avg":string[][], "Ipk_Avg":string[][], "Report_Ref":refnum<class "NI_report.lvclass">, "User Name":string, "Temp_Sheet":string[][]}
  T2 = typedef "Datalog Cluster Array.ctl" = T3[]
  T3 = typedef "Datalog Bundle Control.ctl" = cluster{"Heat":dbl, "WT1800 Functions":T4, "WT1800 Averages":T5, "WT1800 Measurements":T6[][], "DSA Functions":T7, "DSA Averages":T8, "DSA Measurements":T9[][], "Initial Time Stamp":timestamp, "Final Time Stamp":timestamp, "Temperature Data":sgl[][]}
  T4 = typedef "WT1800 Functions.ctl" = cluster{"Channel":string, "Vrms":string, "Power":string, "Vpkpk":string, "Ipkpk":string, "Vpkpk":string}[]
  T5 = typedef "WT1800 Measurements.ctl" = T6[]
  T6 = typedef "WT1800 Readings.ctl" = cluster{"Vrms":sgl, "Irms":sgl, "Power":sgl, "Vpkpk":sgl, "Ipkpk":sgl}
  T7 = typedef "DSA Functions.ctl" = cluster{"Channel":string, "Vrms":string, "Vdc":string, "Vpk+":string, "Vpk-":string, "Vpkpk":string}[]
  T8 = typedef "DSA Measurements.ctl" = T9[]
  T9 = typedef "DSA Readings.ctl" = cluster{"Vrms":sgl, "Vdc":sgl, "Vpk+":sgl, "Vpk-":sgl, "Vpkpk":sgl}
  T10 = typedef "Settings Control.ctl" = cluster{"Supply Voltage [Vdc]":sgl, "Max Supply Current [Idc]":sgl, "Settling Delay":dbl, "Temp Criteria":sgl, "Voltage Steps [Vrms]":sgl[], "User Notes":string, "Config Wave File Path":path, "Config Voltage [Vrms]":sgl, "Channel Configuration List":T11, "User Gains":T14, "Gains":T14, "Gain Array":T15, "Wave File Path 1":path, "Wave File Path 2":path, "Wave File Path 3":path, "Wave File Path 4":path, "Range":bool, "CF":bool}
  T11 = typedef "Channel Configuration List.ctl" = cluster{"Channel Configuration Cluster":T12, "Channel Configuration Cluster 2":T12, "Channel Configuration Cluster 3":T12, "Channel Configuration Cluster 4":T12, "Channel Configuration Cluster 5":T12, "Channel Configuration Cluster 6":T12, "Channel Configuration Cluster 7":T12, "Channel Configuration Cluster 8":T12, "Channel Configuration Cluster 9":T12, "Channel Configuration Cluster 10":T13, "Channel Configuration Cluster 11":T13, "Channel Configuration Cluster 12":T13, "Channel Configuration Cluster 13":T13, "Channel Configuration Cluster 14":T13, "Channel Configuration Cluster 15":T13, "Channel Configuration Cluster 16":T13, "Channel Configuration Cluster 17":T13}
  T12 = typedef "Channel Configuration Cluster.ctl" = cluster{"Input":enum16{"---", "1", "1 AVG", "2", "2 AVG", "3", "3 AVG", "4", "4 AVG"}, "Enable":bool, "User Notes":string, "Voltage Range":dbl, "Current Range":dbl}
  T13 = typedef "Channel Configuration Cluster High Current.ctl" = cluster{"Input":enum16{"---", "1", "1 AVG", "2", "2 AVG", "3", "3 AVG", "4", "4 AVG"}, "Enable":bool, "User Notes":string, "Voltage Range":dbl, "Current Range":dbl}
  T14 = typedef "Gain Averages.ctl" = cluster{"Gain 1":dbl, "Gain 2":dbl, "Gain 3":dbl, "Gain 4":dbl, "Gain 5":dbl, "Gain 6":dbl}
  T15 = typedef "Gain Array.ctl" = cluster{"Gain 1":dbl, "Gain 2":dbl, "Gain 3":dbl, "Gain 4":dbl, "Gain 5":dbl, "Gain 6":dbl, "Gain 7":dbl, "Gain 8":dbl, "Gain 9":dbl, "Gain 10":dbl, "Gain 11":dbl, "Gain 12":dbl, "Gain 13":dbl, "Gain 14":dbl, "Gain 15":dbl, "Gain 16":dbl, "Gain 17":dbl}
  T16 = typedef "Select_Data.ctl" = cluster{"Vrms Data":bool, "Vpkpk Data":bool, "Irms Data":bool, "Power Data":bool, "Ipkpk Data":bool, "Temp Data":bool}
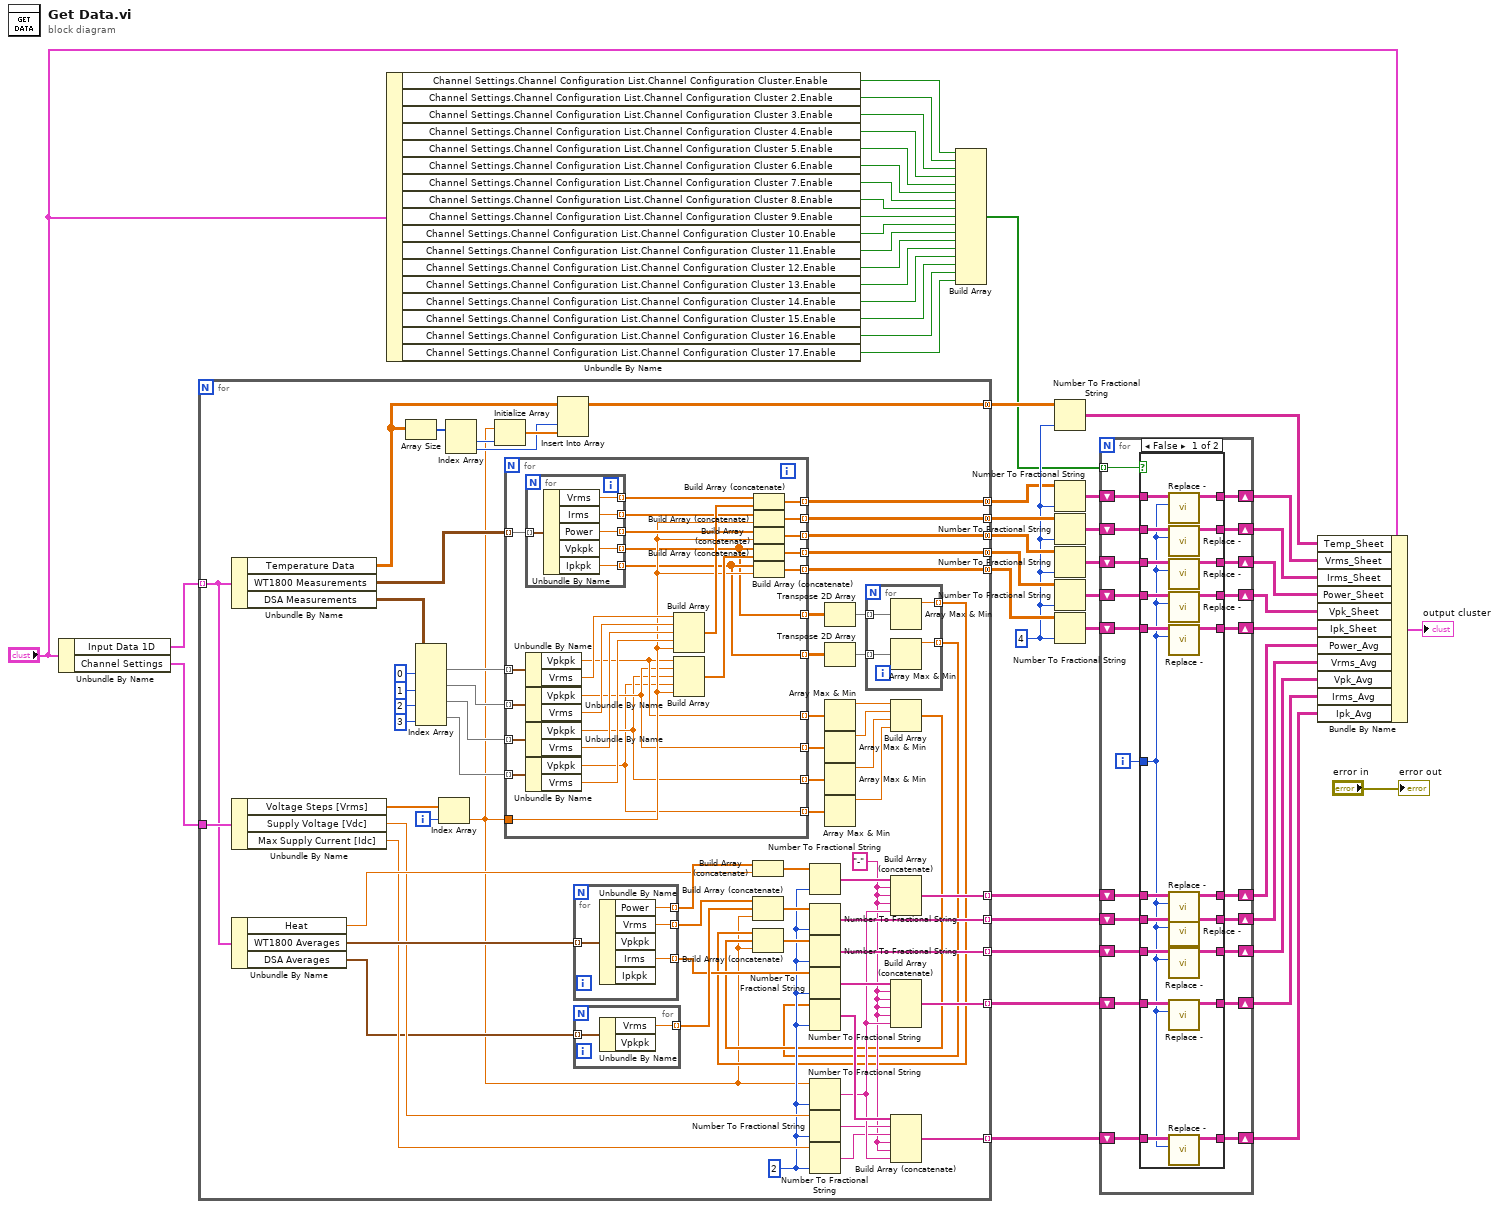
[diagram p0: block diagram]
diagram:
  w43 = i16 4 ("precision (6)")
  n1 = Unbundle By Name("?") -> ("Input Data 1D"=w47:T2, "Channel Settings"=w46:T10)
  n2 = for {
    tunnel: [w117] -> w50 mode=concatenating
    tunnel: [w116] -> w49 mode=concatenating
    tunnel: [w115] -> w48 mode=concatenating
    tunnel: w47 -> [w106] mode=indexing
    tunnel: [w111] -> w1 mode=concatenating
    tunnel: [w110] -> w51 mode=concatenating
    tunnel: w46 -> [w108]
    tunnel: [w100] -> w13 mode=indexing
    tunnel: [w95] -> w12 mode=indexing
    tunnel: [w93] -> w11 mode=indexing
    tunnel: [w90] -> w10 mode=indexing
    tunnel: [w88] -> w9 mode=indexing
    tunnel: [w53] -> w42 mode=concatenating
    i -> [w98]
    w75 = i16 2 ("precision (6)")
    w74 = "-" ("Heat")
    n3 = Unbundle By Name(w106) -> ("Temperature Data"=w54:sgl[][], "WT1800 Measurements"=w86:T6[][], "DSA Measurements"=w109:T9[][])
    n4 = Unbundle By Name(w108) -> ("Voltage Steps [Vrms]"=w107:sgl[], "Supply Voltage [Vdc]"=w85:sgl, "Max Supply Current [Idc]"=w84:sgl)
    n5 = Unbundle By Name(w106) -> ("Heat"=w103:dbl, "WT1800 Averages"=w105:T5, "DSA Averages"=w80:T8)
    n6 = Array Size(array=w54) -> (size(s)=w58:i32[])
    n7 = Index Array(array=w109, index (col) #1=0 ("disabled index (col)"), index (col) #2=1 ("index (col)"), index (col) #3=2 ("index (col)"), index (col) #4=3 ("index (col)")) -> (element #1=w113:T9[], element #2=w112:T9[], element #3=w77:T9[], element #4=w76:T9[])  [unwired: 4 in]
    n8 = Index Array(array=w107, index=w98) -> (element=w52:sgl)
    n9 = Index Array(array=w58) -> (element #1=w57:i32, element #2=w55:i32)  [unwired: 2 in]
    n10 = Initialize Array(w52, w57) -> (w56:sgl[])
    n11 = for {
      tunnel: w86 -> [w153] mode=indexing
      tunnel: [w136] -> w117 mode=indexing
      tunnel: [w146] -> w116 mode=indexing
      tunnel: [w135] -> w115 mode=indexing
      tunnel: w113 -> [w152] mode=indexing
      tunnel: w112 -> [w151] mode=indexing
      tunnel: [w145] -> w111 mode=indexing
      tunnel: [w138] -> w110 mode=indexing
      tunnel: w52 -> [w134]
      tunnel: w77 -> [w143] mode=indexing
      tunnel: w76 -> [w142] mode=indexing
      tunnel: [w133] -> w67 mode=indexing
      tunnel: [w132] -> w66 mode=indexing
      tunnel: [w131] -> w65 mode=indexing
      tunnel: [w130] -> w64 mode=indexing
      tunnel: [w129] -> w63 mode=indexing
      tunnel: [w128] -> w62 mode=indexing
      n12 = for {
        tunnel: w153 -> [w159] mode=indexing
        tunnel: [w158] -> w148 mode=indexing
        tunnel: [w157] -> w139 mode=indexing
        tunnel: [w156] -> w137 mode=indexing
        tunnel: [w155] -> w132 mode=indexing
        tunnel: [w154] -> w133 mode=indexing
        n13 = Unbundle By Name(w159) -> ("Vrms"=w158:sgl, "Irms"=w157:sgl, "Power"=w156:sgl, "Vpkpk"=w155:sgl, "Ipkpk"=w154:sgl)
      }
      n14 = Unbundle By Name(w152) -> ("Vpkpk"=w131:sgl, "Vrms"=w150:sgl)
      n15 = Unbundle By Name(w151) -> ("Vpkpk"=w130:sgl, "Vrms"=w149:sgl)
      n16 = Unbundle By Name(w143) -> ("Vpkpk"=w129:sgl, "Vrms"=w141:sgl)
      n17 = Unbundle By Name(w142) -> ("Vpkpk"=w128:sgl, "Vrms"=w140:sgl)
      n18 = Build Array(w150, w149, w141, w140, w134) -> (w144:sgl[])
      n19 = Build Array(w131, w130, w129, w128, w134) -> (w147:sgl[])
      n20 = Build Array (concatenate)(w148, w144) -> (w145:sgl[])
      n21 = Build Array (concatenate)(w139, w134) -> (w138:sgl[])
      n22 = Build Array (concatenate)(w137, w134) -> (w136:sgl[])
      n23 = Build Array (concatenate)(w132, w147) -> (w146:sgl[])
      n24 = Build Array (concatenate)(w133, w134) -> (w135:sgl[])
    }
    n25 = Insert Into Array(array=w54, index (col)=w55, new element=w56) -> (w53:sgl[][])  [unwired: 1 in]
    n26 = for {
      tunnel: w105 -> [w127] mode=indexing
      tunnel: [w124] -> w104 mode=indexing
      tunnel: [w126] -> w99 mode=indexing
      tunnel: [w125] -> w92 mode=indexing
      n27 = Unbundle By Name(w127) -> ("Power"=w124:sgl, "Vrms"=w126:sgl, "Irms"=w125:sgl)  [unwired: 2 out]
    }
    n28 = for {
      tunnel: [w123] -> w97 mode=indexing
      tunnel: w80 -> [w122] mode=indexing
      n29 = Unbundle By Name(w122) -> ("Vrms"=w123:sgl)  [unwired: 1 out]
    }
    n30 = Build Array (concatenate)(w104, w103) -> (w102:dbl[])
    n31 = Build Array (concatenate)(w99, w97, w52) -> (w96:sgl[])
    n32 = Number To Fractional String(number=w102, precision (6)=w75) -> (F-format string=w101:string[])  [unwired: 2 in]
    n33 = Number To Fractional String(number=w96, precision (6)=w75) -> (F-format string=w95:string[])  [unwired: 2 in]
    n34 = Number To Fractional String(number=w92, precision (6)=w75) -> (F-format string=w91:string[])  [unwired: 2 in]
    n35 = Number To Fractional String(number=w52, precision (6)=w75) -> (F-format string=w87:string)  [unwired: 2 in]
    n36 = Number To Fractional String(number=w85, precision (6)=w75) -> (F-format string=w83:string)  [unwired: 2 in]
    n37 = Number To Fractional String(number=w84, precision (6)=w75) -> (F-format string=w82:string)  [unwired: 2 in]
    n38 = Transpose 2D Array(2D array=w66) -> (transposed array=w73:sgl[][])
    n39 = Transpose 2D Array(2D array=w67) -> (transposed array=w72:sgl[][])
    n40 = Array Max & Min(array=w65) -> (max value=w71:sgl)  [unwired: 3 out]
    n41 = Array Max & Min(array=w64) -> (max value=w68:sgl)  [unwired: 3 out]
    n42 = Array Max & Min(array=w63) -> (max value=w69:sgl)  [unwired: 3 out]
    n43 = Array Max & Min(array=w62) -> (max value=w70:sgl)  [unwired: 3 out]
    n44 = for {
      tunnel: w73 -> [w121] mode=indexing
      tunnel: [w120] -> w61 mode=indexing
      tunnel: w72 -> [w119] mode=indexing
      tunnel: [w118] -> w59 mode=indexing
      n45 = Array Max & Min(array=w121) -> (max value=w120:sgl)  [unwired: 3 out]
      n46 = Array Max & Min(array=w119) -> (max value=w118:sgl)  [unwired: 3 out]
    }
    n47 = Number To Fractional String(number=w59, precision (6)=w75) -> (F-format string=w89:string[])  [unwired: 2 in]
    n48 = Build Array(w71, w68, w69, w70) -> (w60:sgl[])
    n49 = Build Array (concatenate)(w61, w60, w52) -> (w94:sgl[])
    n50 = Number To Fractional String(number=w94, precision (6)=w75) -> (F-format string=w93:string[])  [unwired: 2 in]
    n51 = Build Array (concatenate)(w101, w74, w74, w74, w87) -> (w100:string[])
    n52 = Build Array (concatenate)(w91, w74, w74, w74, w74, w87) -> (w90:string[])
    n53 = Build Array (concatenate)(w89, w83, w82, w74, w74, w87) -> (w88:string[])
  }
  n54 = Unbundle By Name("?") -> ("Channel Settings.Channel Configuration List.Channel Configuration Cluster.Enable"=w36:bool, "Channel Settings.Channel Configuration List.Channel Configuration Cluster 2.Enable"=w35:bool, "Channel Settings.Channel Configuration List.Channel Configuration Cluster 3.Enable"=w34:bool, "Channel Settings.Channel Configuration List.Channel Configuration Cluster 4.Enable"=w33:bool, "Channel Settings.Channel Configuration List.Channel Configuration Cluster 5.Enable"=w32:bool, "Channel Settings.Channel Configuration List.Channel Configuration Cluster 6.Enable"=w31:bool, "Channel Settings.Channel Configuration List.Channel Configuration Cluster 7.Enable"=w30:bool, "Channel Settings.Channel Configuration List.Channel Configuration Cluster 8.Enable"=w29:bool, "Channel Settings.Channel Configuration List.Channel Configuration Cluster 9.Enable"=w28:bool, "Channel Settings.Channel Configuration List.Channel Configuration Cluster 10.Enable"=w27:bool, "Channel Settings.Channel Configuration List.Channel Configuration Cluster 11.Enable"=w26:bool, "Channel Settings.Channel Configuration List.Channel Configuration Cluster 12.Enable"=w25:bool, "Channel Settings.Channel Configuration List.Channel Configuration Cluster 13.Enable"=w24:bool, "Channel Settings.Channel Configuration List.Channel Configuration Cluster 14.Enable"=w23:bool, "Channel Settings.Channel Configuration List.Channel Configuration Cluster 15.Enable"=w22:bool, "Channel Settings.Channel Configuration List.Channel Configuration Cluster 16.Enable"=w21:bool, "Channel Settings.Channel Configuration List.Channel Configuration Cluster 17.Enable"=w20:bool)
  n55 = Build Array(w36, w35, w34, w33, w32, w31, w30, w29, w28, w27, w26, w25, w24, w23, w22, w21, w20) -> (w19:bool[])
  n56 = Number To Fractional String(number=w42, precision (6)=w43) -> (F-format string=w3:string[][])  [unwired: 2 in]
  n57 = Number To Fractional String(number=w1, precision (6)=w43) -> (F-format string=w41:string[][])  [unwired: 2 in]
  n58 = Number To Fractional String(number=w51, precision (6)=w43) -> (F-format string=w40:string[][])  [unwired: 2 in]
  n59 = Number To Fractional String(number=w50, precision (6)=w43) -> (F-format string=w39:string[][])  [unwired: 2 in]
  n60 = Number To Fractional String(number=w49, precision (6)=w43) -> (F-format string=w38:string[][])  [unwired: 2 in]
  n61 = Number To Fractional String(number=w48, precision (6)=w43) -> (F-format string=w37:string[][])  [unwired: 2 in]
  n62 = for {
    tunnel: w19 -> [w176] mode=indexing
    shift-right: [w174] -> w18
    shift-left: w41 -> [w181]
    shift-right: [w173] -> w17
    shift-left: w40 -> [w180]
    shift-right: [w172] -> w16
    shift-left: w39 -> [w179]
    shift-right: [w171] -> w15
    shift-left: w38 -> [w178]
    shift-right: [w170] -> w14
    shift-left: w37 -> [w177]
    shift-right: [w164] -> w8
    shift-left: w13 -> [w169]
    shift-right: [w163] -> w7
    shift-left: w12 -> [w168]
    shift-right: [w162] -> w6
    shift-left: w11 -> [w167]
    shift-right: [w161] -> w5
    shift-left: w10 -> [w166]
    shift-right: [w160] -> w4
    shift-left: w9 -> [w165]
    i -> [w175]
    n63 = case shown="False" w176 {
      tunnel: w181 -> [w202 w212]
      tunnel: w180 -> [w201 w211]
      tunnel: w179 -> [w200 w210]
      tunnel: w178 -> [w199 w209]
      tunnel: w177 -> [w198 w208]
      tunnel: w175 -> [w192 _]
      tunnel: [w191 w212] -> w174
      tunnel: [w190 w211] -> w173
      tunnel: [w189 w210] -> w172
      tunnel: [w188 w209] -> w171
      tunnel: [w187 w208] -> w170
      tunnel: w169 -> [w197 w207]
      tunnel: w168 -> [w196 w206]
      tunnel: w167 -> [w195 w205]
      tunnel: w166 -> [w194 w204]
      tunnel: w165 -> [w193 w203]
      tunnel: [w186 w207] -> w164
      tunnel: [w185 w206] -> w163
      tunnel: [w184 w205] -> w162
      tunnel: [w183 w204] -> w161
      tunnel: [w182 w203] -> w160
      frame False {
        n64 = call "Replace -.vi"("Numeric"=w192, "Array in"=w202) -> ("Array out"=w191:string[][])  [unwired: 9 in]
        n65 = call "Replace -.vi"("Numeric"=w192, "Array in"=w201) -> ("Array out"=w190:string[][])  [unwired: 9 in]
        n66 = call "Replace -.vi"("Numeric"=w192, "Array in"=w200) -> ("Array out"=w189:string[][])  [unwired: 9 in]
        n67 = call "Replace -.vi"("Numeric"=w192, "Array in"=w199) -> ("Array out"=w188:string[][])  [unwired: 9 in]
        n68 = call "Replace -.vi"("Numeric"=w192, "Array in"=w198) -> ("Array out"=w187:string[][])  [unwired: 9 in]
        n69 = call "Replace -.vi"("Numeric"=w192, "Array in"=w197) -> ("Array out"=w186:string[][])  [unwired: 9 in]
        n70 = call "Replace -.vi"("Numeric"=w192, "Array in"=w196) -> ("Array out"=w185:string[][])  [unwired: 9 in]
        n71 = call "Replace -.vi"("Numeric"=w192, "Array in"=w195) -> ("Array out"=w184:string[][])  [unwired: 9 in]
        n72 = call "Replace -.vi"("Numeric"=w192, "Array in"=w194) -> ("Array out"=w183:string[][])  [unwired: 9 in]
        n73 = call "Replace -.vi"("Numeric"=w192, "Array in"=w193) -> ("Array out"=w182:string[][])  [unwired: 9 in]
      }
      frame True {
      }
    }
  }
  n74 = Bundle By Name(cluster="?", "Temp_Sheet"=w3, "Vrms_Sheet"=w18, "Irms_Sheet"=w17, "Power_Sheet"=w16, "Vpk_Sheet"=w15, "Ipk_Sheet"=w14, "Power_Avg"=w8, "Vrms_Avg"=w7, "Vpk_Avg"=w6, "Irms_Avg"=w5, "Ipk_Avg"=w4) -> (→"output cluster":T1)
  "error out" <- "error in"
